vi "TestFFTfunction.vi"() -> ()   [LabVIEW 2018]
uses:
  General Libraries/Photon Filtering.lvlib
  <vilib>/Analysis/NI_AALBase.lvlib
  <vilib>/Analysis/baseanly.llb/Real Outer Product.vi
  General Libraries/myFFT.lvlib
panel:
  in  "Tab Control":enum32{"simulate result", "parameters"}(tab)
  out "fft":dbl[][](graph)
  out "image":dbl[][](graph)
  out "filtered image":dbl[][](graph)
  in  "Mask ON":bool
  out "fft cluster":T1
  in  "Nlines":i32=1024
  in  "df":dbl=1.0 format="%#_13g"
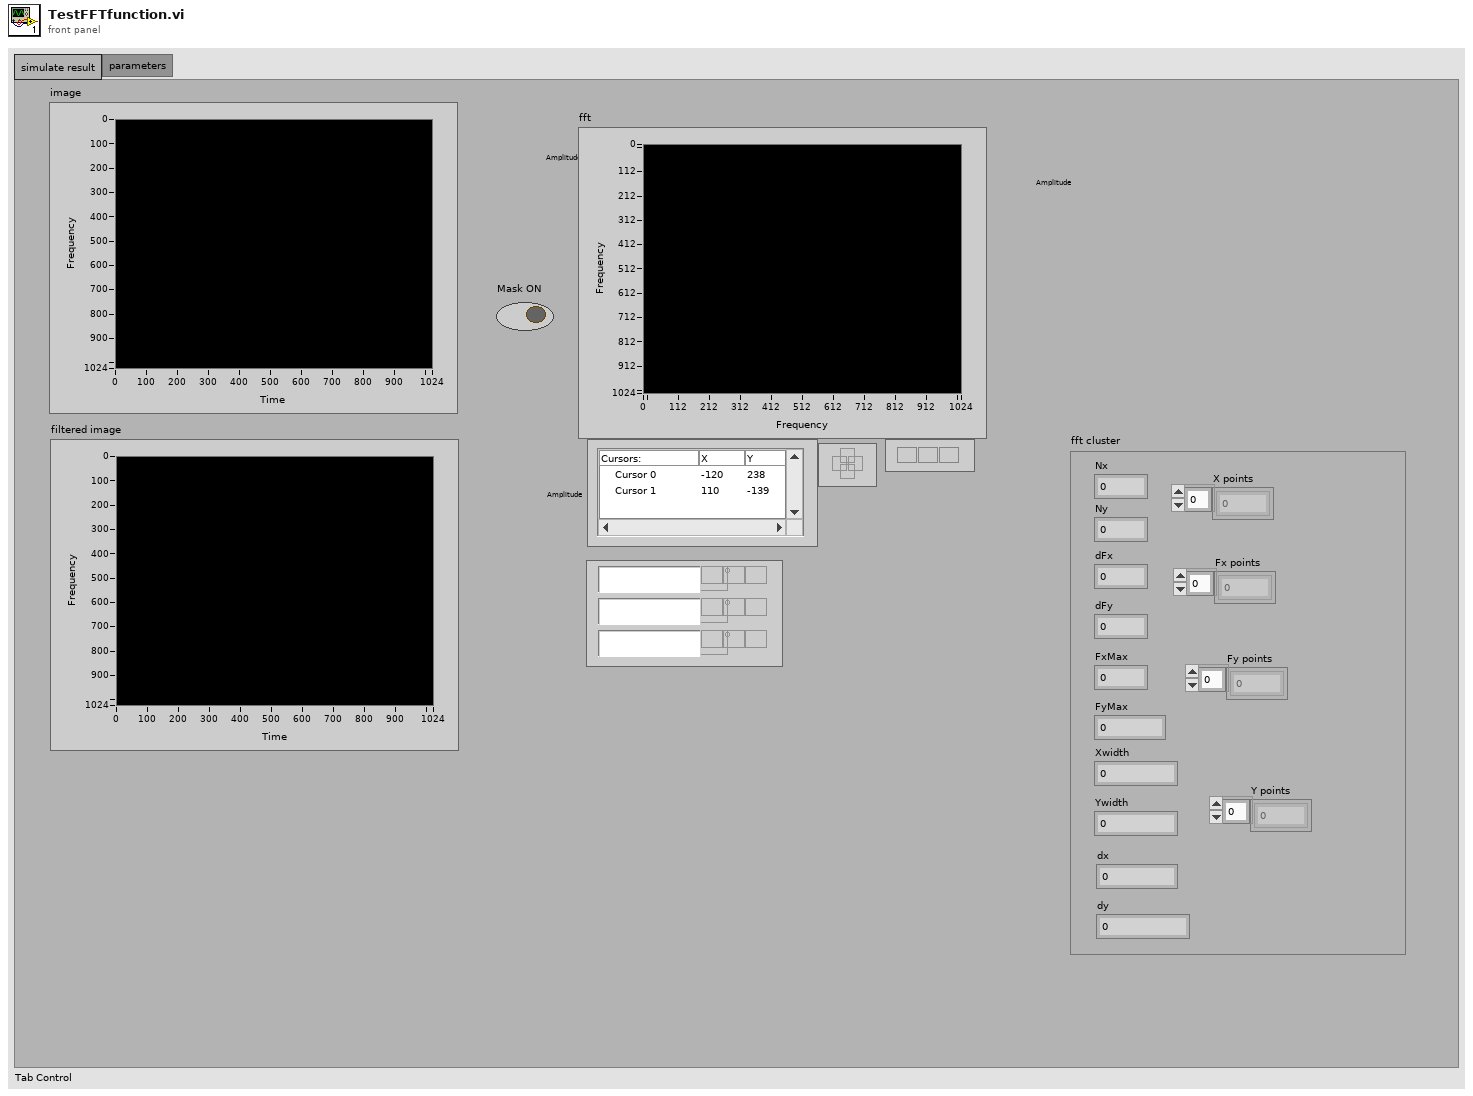
[diagram p1: front panel]
types:
  T1 = cluster{"dFx":dbl, "dFy":dbl, "Nx":i32, "Ny":i32, "FxMax":dbl, "FyMax":dbl, "Xwidth":dbl, "Ywidth":dbl, "dx":dbl, "dy":dbl, "Fx points":dbl[], "X points":dbl[], "Y points":dbl[], "Fy points":dbl[]}
  T2 = typedef "NI_Matrix.lvlib/RealMatrix.ctl" = dbl[][]
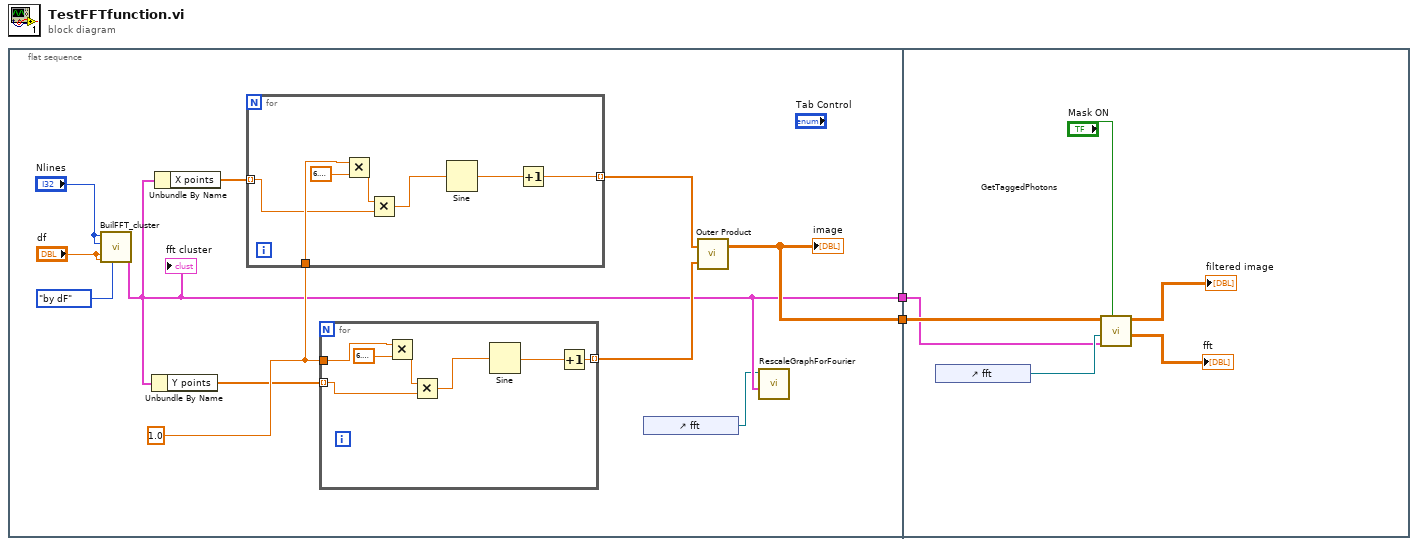
[diagram p0: block diagram]
diagram:
  n1 = flat-sequence {
    tunnel: [w12] -> w2
    tunnel: [w4] -> w1
    tunnel: w2 -> [w33]
    tunnel: w1 -> [w28]
    frame #0 {
      w8 = 1.0 ("y")
      n2 = call "BuilFFT_cluster.vi"("Enum"=enum16{"by dF", "by dX"}."by dF", "input Y"="df", "input X"="df", "Ny"="Nlines", "Nx"="Nlines") -> ("fft cluster"=w4:T1)  [unwired: 6 in]
      "fft cluster" <- w4
      n3 = Unbundle By Name(w4) -> ("Y points"=w6:dbl[])
      n4 = Unbundle By Name(w4) -> ("X points"=w9:dbl[])
      n5 = for {
        tunnel: w9 -> [w16] mode=indexing
        tunnel: w8 -> [w17]
        tunnel: [w14] -> w7 mode=indexing
        n6 = Multiply(x=w17, y=6.283185307179586) -> (x*y=w19:dbl)
        n7 = Multiply(x=w19, y=w16) -> (x*y=w18:dbl)
        n8 = Sine(x=w18) -> (sin(x)=w15:dbl)
        n9 = Increment(x=w15) -> (x+1=w14:dbl)
      }
      n10 = for {
        tunnel: [w24] -> w13 mode=indexing
        tunnel: w8 -> [w22]
        tunnel: w6 -> [w21] mode=indexing
        n11 = Multiply(x=w22, y=6.283185307179586) -> (x*y=w26:dbl)
        n12 = Multiply(x=w26, y=w21) -> (x*y=w25:dbl)
        n13 = Sine(x=w25) -> (sin(x)=w23:dbl)
        n14 = Increment(x=w23) -> (x+1=w24:dbl)
      }
      n15 = control-ref of="fft"() -> (w3:refnum<vi>)
      n16 = call-poly <vilib>:"Outer Product.vi"("Y Vector"=w13, "X Vector"=w7) -> ("Outer Product"=w12:T2)  [unwired: 1 out]
      "image" <- w12
      n17 = call "RescaleGraphForFourier.vi"("fft reference"=w3, "fft cluster"=w4) -> ()  [unwired: 9 in]
    }
    frame #1 {
      n18 = control-ref of="fft"() -> (w32:refnum<vi>)
      n19 = call "GetTaggedPhotons.vi"("screen status"="Mask ON", "fft cluster"=w28, "FFT reference"=w32, "double precision float"=w33) -> ("FFT modulous"=→"fft":dbl[][], "tagged photons"=→"filtered image":dbl[][])  [unwired: 4 in, 2 out]
    }
  }
